vi "raster_scan_ground_shutter.vi"() -> ()   [LabVIEW 2013] (continued)
  out "Spectra":cluster{"X":dbl, "Y":dbl}[](graph)=[{"X"=497.2298226599585, "Y"=0.9725975182005102}, {"X"=498.51538166101153, "Y"=0.9728067925850153}, {"X"=499.8006653114716, "Y"=0.9747721051033233}, {"X"=501.08567369979005, "Y"=0.9751655628735649}, {"X"=502.37040691438784, "Y"=0.9732612176842215}, {"X"=503.65486504364054, "Y"=0.9746414011783826}, {"X"=504.9390481758954, "Y"=0.9742385776980085}, {"X"=506.2229563994542, "Y"=0.9735153291445955}, {"X"=507.50658980258396, "Y"=0.9733135229509433}, {"X"=508.7899484735106, "Y"=0.9744504839918318}, {"X"=510.0730325004275, "Y"=0.9766044345160604}, {"X"=511.3558419714845, "Y"=0.9750567839983721}, {"X"=512.6383769748013, "Y"=0.971673355532271}, {"X"=513.92063759845, "Y"=0.9740526614709577}, {"X"=515.2026239304761, "Y"=0.974130815359634}, {"X"=516.484336058878, "Y"=0.9752353326241979}, {"X"=517.7657740716236, "Y"=0.9733187917634595}, {"X"=519.0469380566371, "Y"=0.9738867743443941}, {"X"=520.3278281018086, "Y"=0.9741291463192384}, {"X"=521.6084442949887, "Y"=0.9739939491908779}, {"X"=522.8887867239932, "Y"=0.9738818697876678}, {"X"=524.1688554765973, "Y"=0.9751365110316095}, {"X"=525.448650640541, "Y"=0.9756894098172196}, {"X"=526.7281723035276, "Y"=0.9755958341013884}, {"X"=528.0074205532212, "Y"=0.9723731001887784}, {"X"=529.286395477245, "Y"=0.9736078210171095}, {"X"=530.5650971631895, "Y"=0.9753577492499681}, {"X"=531.8435256986106, "Y"=0.9756076345965283}, {"X"=533.1216811710165, "Y"=0.9749519370844743}, {"X"=534.3995636678867, "Y"=0.9737182292893943}, {"X"=535.6771732766625, "Y"=0.9731227772162603}, {"X"=536.954510084748, "Y"=0.9743263327011618}, {"X"=538.2315741795014, "Y"=0.9748905035101719}, {"X"=539.5083656482575, "Y"=0.9726015732101311}, {"X"=540.7848845783033, "Y"=0.9742346225867319}, {"X"=542.061131056891, "Y"=0.973702680791654}, {"X"=543.3371051712381, "Y"=0.9745816372249786}, {"X"=544.6128070085233, "Y"=0.9746140975084203}, {"X"=545.888236655888, "Y"=0.9745470905602152}, {"X"=547.1633942004373, "Y"=0.9740537792906223}, {"X"=548.438279729239, "Y"=0.9704166842457509}, {"X"=549.7128933293197, "Y"=0.9754447594924198}, {"X"=550.987235087676, "Y"=0.9748748689433028}, {"X"=552.261305091261, "Y"=0.9747804617231326}, {"X"=553.5351034269949, "Y"=0.9754642257486512}, {"X"=554.8086301817569, "Y"=0.9736484025754294}, {"X"=556.0818854423965, "Y"=0.9748432686352313}, {"X"=557.3548692957187, "Y"=0.9719628762042646}, {"X"=558.6275818284925, "Y"=0.9746558278490033}, {"X"=559.9000231274539, "Y"=0.9738137515041241}, {"X"=561.1721932793001, "Y"=0.9716527613161314}, {"X"=562.4440923706871, "Y"=0.974021060448881}, {"X"=563.7157204882404, "Y"=0.9728545916304719}, {"X"=564.9870777185446, "Y"=0.9732879649303774}, {"X"=566.2581641481513, "Y"=0.9744530162766258}, {"X"=567.5289798635712, "Y"=0.974627123784301}, {"X"=568.7995249512783, "Y"=0.9725287766595139}, {"X"=570.0697994977114, "Y"=0.9726663869699587}, {"X"=571.339803589273, "Y"=0.974955727849392}, {"X"=572.6095373123283, "Y"=0.9735543225094384}, {"X"=573.8790007532059, "Y"=0.9724127620578475}, {"X"=575.148193998193, "Y"=0.9740209723716318}, {"X"=576.4171171335469, "Y"=0.9735745739854244}, {"X"=577.6857702454895, "Y"=0.9736808497462064}, {"X"=578.9541534201954, "Y"=0.973725135201695}, {"X"=580.2222667438133, "Y"=0.9722570169385129}, {"X"=581.4901103024504, "Y"=0.9761561614512213}, {"X"=582.7576841821772, "Y"=0.9745066084652275}, {"X"=584.0249884690273, "Y"=0.9721193991121173}, {"X"=585.2920232489998, "Y"=0.9730164211590435}, {"X"=586.5587886080565, "Y"=0.9744353227462825}, {"X"=587.8252846321227, "Y"=0.9740001461801483}, {"X"=589.0915114070889, "Y"=0.9730116363864676}, {"X"=590.3574690188022, "Y"=0.9727604590195043}, {"X"=591.6231575530794, "Y"=0.9741329926815703}, {"X"=592.8885770957004, "Y"=0.9715013368639458}, {"X"=594.1537277324082, "Y"=0.9749212992460508}, {"X"=595.4186095489069, "Y"=0.9746155414778752}, {"X"=596.6832226308679, "Y"=0.9733153658733915}, {"X"=597.9475670639238, "Y"=0.9738269855570807}, {"X"=599.2116429336721, "Y"=0.9727047693027512}, {"X"=600.4754503256718, "Y"=0.9723284099559123}, {"X"=601.7389893254467, "Y"=0.9739548965405067}, {"X"=603.0022600184864, "Y"=0.9753519803682732}, {"X"=604.2652624902432, "Y"=0.9745724974660718}, {"X"=605.5279968261262, "Y"=0.9739205053321395}, {"X"=606.790463111523, "Y"=0.9733144490021569}, {"X"=608.0526614317708, "Y"=0.9736048889225003}, {"X"=609.3145918721773, "Y"=0.9737789504525353}, {"X"=610.5762545180146, "Y"=0.9755778166852583}, {"X"=611.8376494545141, "Y"=0.9730244273499707}, {"X"=613.0987767668724, "Y"=0.9728226921337769}, {"X"=614.3596365402559, "Y"=0.9752868467363005}, {"X"=615.6202288597873, "Y"=0.9735172698359681}, {"X"=616.8805538105571, "Y"=0.973124505522509}, {"X"=618.1406114776187, "Y"=0.9760376947254987}, {"X"=619.4004019459886, "Y"=0.9749446586217881}, {"X"=620.659925300649, "Y"=0.9727135962087332}, {"X"=621.9191816265427, "Y"=0.9769047701336491}, {"X"=623.1781710085843, "Y"=0.9737059369513906}, {"X"=624.4368935316431, "Y"=0.9730367708590156}, {"X"=625.6953492805558, "Y"=0.973595493502758}, {"X"=626.9535383401242, "Y"=0.9741996880818808}, {"X"=628.2114607951178, "Y"=0.9737205194986359}, {"X"=629.4691167302606, "Y"=0.9749579037936418}, {"X"=630.7265062302503, "Y"=0.9743079192507641}, {"X"=631.9836293797415, "Y"=0.9752794157731268}, {"X"=633.2404862633583, "Y"=0.9724798256913757}, {"X"=634.4970769656837, "Y"=0.9740631998947202}, {"X"=635.7534015712725, "Y"=0.9728994698167882}, {"X"=637.0094601646339, "Y"=0.9739938061766921}, {"X"=638.2652528302488, "Y"=0.9725288232542131}, {"X"=639.5207796525636, "Y"=0.9736153995992328}, {"X"=640.7760407159792, "Y"=0.9729825812921996}, {"X"=642.0310361048703, "Y"=0.9744619006373575}, {"X"=643.2857659035727, "Y"=0.9730632124324957}, {"X"=644.5402301963852, "Y"=0.9721840737194735}, {"X"=645.7944290675744, "Y"=0.974009871166903}, {"X"=647.0483626013629, "Y"=0.972528548755031}, {"X"=648.3020308819501, "Y"=0.9722772695955144}, {"X"=649.5554339934918, "Y"=0.976397196845756}, {"X"=650.8085720201068, "Y"=0.9735361483405925}, {"X"=652.0614450458858, "Y"=0.9743662972168945}, {"X"=653.3140531548762, "Y"=0.9733556726469628}, {"X"=654.5663964310929, "Y"=0.973308883274387}, {"X"=655.8184749585181, "Y"=0.9729671339680315}, {"X"=657.0702888210908, "Y"=0.9735267285897199}, {"X"=658.321838102726, "Y"=0.9736835283965779}, {"X"=659.5731228872934, "Y"=0.9724850110082932}, {"X"=660.8241432586319, "Y"=0.9768246153401708}, {"X"=662.0748993005419, "Y"=0.9747368444941559}, {"X"=663.3253910967932, "Y"=0.9748671054129099}, {"X"=664.5756187311121, "Y"=0.9712450801505587}, {"X"=665.8255822872012, "Y"=0.9733016295621294}, {"X"=667.0752818487133, "Y"=0.9751572607097476}, {"X"=668.3247174992814, "Y"=0.9736732199722962}, {"X"=669.5738893224913, "Y"=0.9714170347757555}, {"X"=670.8227974018998, "Y"=0.9744672290673195}, {"X"=672.0714418210257, "Y"=0.9735008611418889}, {"X"=673.3198226633544, "Y"=0.9753387615125017}, {"X"=674.5679400123306, "Y"=0.973086840492722}, {"X"=675.8157939513727, "Y"=0.9741838697202261}, {"X"=677.063384563856, "Y"=0.973529280298374}, {"X"=678.3107119331249, "Y"=0.9755250682367654}, {"X"=679.5577761424901, "Y"=0.9746411843678233}, {"X"=680.8045772752221, "Y"=0.9738103562180661}, {"X"=682.0511154145598, "Y"=0.9736968628203867}, {"X"=683.2973906437047, "Y"=0.9712589511537898}, {"X"=684.5434030458239, "Y"=0.9752582378141089}, {"X"=685.7891527040539, "Y"=0.976782251150417}, {"X"=687.0346397014858, "Y"=0.9731820071149043}, {"X"=688.2798641211891, "Y"=0.9733579906581664}, {"X"=689.5248260461898, "Y"=0.9744816274791854}, {"X"=690.769525559477, "Y"=0.9737516724400619}, {"X"=692.0139627440117, "Y"=0.9756854529656466}, {"X"=693.2581376827137, "Y"=0.9752736616888705}, {"X"=694.5020504584725, "Y"=0.9747129818582982}, {"X"=695.7457011541385, "Y"=0.9725964644867655}, {"X"=696.9890898525315, "Y"=0.9719206032188724}, {"X"=698.2322166364349, "Y"=0.975109207481176}, {"X"=699.4750815885972, "Y"=0.973770575651193}, {"X"=700.7176847917299, "Y"=0.9719288969600468}, {"X"=701.9600263285121, "Y"=0.9733333355442666}, {"X"=703.202106281586, "Y"=0.974777916241537}, {"X"=704.4439247335613, "Y"=0.9735484419792764}, {"X"=705.685481767011, "Y"=0.9717628831069969}, {"X"=706.9267774644752, "Y"=0.974585085670975}, {"X"=708.1678119084597, "Y"=0.9726989197644662}, {"X"=709.4085851814332, "Y"=0.9726006427385325}, {"X"=710.6490973658297, "Y"=0.9733097555076762}, {"X"=711.8893485440507, "Y"=0.9737219810572065}, {"X"=713.1293387984609, "Y"=0.9733159043764248}, {"X"=714.3690682113926, "Y"=0.974995019683123}, {"X"=715.6085368651409, "Y"=0.9744552200280534}, {"X"=716.8477448419642, "Y"=0.9728058762546018}, {"X"=718.0866922240972, "Y"=0.9737322943321336}, {"X"=719.3253790937289, "Y"=0.9735161803203743}, {"X"=720.5638055330157, "Y"=0.9730407067730923}, {"X"=721.8019716240839, "Y"=0.9709235684588909}, {"X"=723.0398774490205, "Y"=0.9745749775668794}, {"X"=724.2775230898802, "Y"=0.9744302526361133}, {"X"=725.5149086286827, "Y"=0.9723284652393392}, {"X"=726.7520341474134, "Y"=0.9753523975377738}, {"X"=727.9888997280249, "Y"=0.9750521852197641}, {"X"=729.2255054524308, "Y"=0.9745820478316395}, {"X"=730.4618514025187, "Y"=0.9742877083296526}, {"X"=731.6979376601308, "Y"=0.9751639925657974}, {"X"=732.933764307081, "Y"=0.976816750584068}, {"X"=734.1693314251528, "Y"=0.974162397219554}, {"X"=735.4046390960863, "Y"=0.9739741725110216}, {"X"=736.6396874015912, "Y"=0.9762852769993037}, {"X"=737.8744764233495, "Y"=0.9766708999836823}, {"X"=739.109006242997, "Y"=0.9753035240381733}, {"X"=740.343276942146, "Y"=0.975790884711858}, {"X"=741.5772886023653, "Y"=0.9766658088688991}, {"X"=742.8110413051957, "Y"=0.9785306717888759}, {"X"=744.0445351321432, "Y"=0.9760682422453827}, {"X"=745.2777701646746, "Y"=0.9780204446669288}, {"X"=746.5107464842309, "Y"=0.9782464109417868}, {"X"=747.7434641722119, "Y"=0.9772647154022579}, {"X"=748.9759233099848, "Y"=0.977692155970407}, {"X"=750.2081239788884, "Y"=0.9788852914399129}, {"X"=751.4400662602164, "Y"=0.9823419830408691}, {"X"=752.6717502352384, "Y"=0.9810201141633521}, {"X"=753.9031759851828, "Y"=0.9833986641137518}, {"X"=755.1343435912498, "Y"=0.9834070429804402}, {"X"=756.365253134605, "Y"=0.9825903876301169}, {"X"=757.5959046963706, "Y"=0.9839529209095583}, {"X"=758.8262983576512, "Y"=0.9813652342798371}, {"X"=760.0564341995022, "Y"=0.9844503443823484}, {"X"=761.2863123029542, "Y"=0.9839336674911496}, {"X"=762.5159327489974, "Y"=0.9850987306074251}, {"X"=763.7452956185957, "Y"=0.9859738872506251}, {"X"=764.9744009926738, "Y"=0.987104856944398}, {"X"=766.2032489521198, "Y"=0.986614152333766}, {"X"=767.4318395777977, "Y"=0.9923688895733606}, {"X"=768.6601729505263, "Y"=0.9903239765936077}, {"X"=769.8882491511001, "Y"=0.989832503713793}, {"X"=771.1160682602751, "Y"=0.9898834352980211}, {"X"=772.3436303587699, "Y"=0.9909275800922739}, {"X"=773.5709355272775, "Y"=0.9922316521951728}, {"X"=774.7979838464516, "Y"=0.9943163001250186}, {"X"=776.0247753969135, "Y"=0.9959180362878817}, {"X"=777.2513102592497, "Y"=0.9979176063076446}, {"X"=778.4775885140167, "Y"=0.997428897906833}, {"X"=779.7036102417335, "Y"=0.999946223134333}, {"X"=780.9293755228872, "Y"=0.9999233980339695}, {"X"=782.1548844379298, "Y"=1.001903497089305}, {"X"=783.3801370672809, "Y"=1.0032164241060768}, {"X"=784.6051334913254, "Y"=1.0017013431572122}, {"X"=785.8298737904138, "Y"=1.0042953210934331}, {"X"=787.0543580448677, "Y"=1.0057069045811273}, {"X"=788.2785863349704, "Y"=1.0040647666748501}, {"X"=789.5025587409746, "Y"=1.0051867459428807}, {"X"=790.7262753430958, "Y"=1.005057036199781}, {"X"=791.9497362215196, "Y"=1.0059360518630067}, {"X"=793.1729414563946, "Y"=1.008461102054222}, {"X"=794.3958911278411, "Y"=1.0087710728267973}, {"X"=795.6185853159403, "Y"=1.0112013829888278}, {"X"=796.8410241007414, "Y"=1.0111463852575098}, {"X"=798.0632075622646, "Y"=1.0110431430825668}, {"X"=799.2851357804917, "Y"=1.0112207906905948}, {"X"=800.5068088353718, "Y"=1.0108210325661546}, {"X"=801.7282268068236, "Y"=1.0109641328064574}, {"X"=802.9493897747267, "Y"=1.0130948150317125}, {"X"=804.1702978189347, "Y"=1.0119276625964746}, {"X"=805.3909510192625, "Y"=1.0117322027094646}, {"X"=806.6113494554919, "Y"=1.0104670902674695}, {"X"=807.8314932073748, "Y"=1.0125669362027019}, {"X"=809.0513823546283, "Y"=1.008923051883943}, {"X"=810.2710169769346, "Y"=1.0076251693882987}, {"X"=811.4903971539436, "Y"=1.0059566148313221}, {"X"=812.7095229652726, "Y"=1.0075916782638574}, {"X"=813.9283944905064, "Y"=1.0041324355776649}, {"X"=815.1470118091908, "Y"=1.0035018727995872}, {"X"=816.3653750008475, "Y"=1.0030209370577858}, {"X"=817.5834841449596, "Y"=0.999972510646731}, {"X"=818.8013393209794, "Y"=0.9982311340973924}, {"X"=820.0189406083226, "Y"=0.9980286387783647}, {"X"=821.2362880863745, "Y"=0.9966341239361585}, {"X"=822.453381834488, "Y"=0.993060330533325}, {"X"=823.6702219319809, "Y"=0.9917217165409767}, {"X"=824.8868084581368, "Y"=0.9904613412583302}, {"X"=826.1031414922085, "Y"=0.9890170518352254}, {"X"=827.3192211134187, "Y"=0.988833927457964}, {"X"=828.5350474009513, "Y"=0.9841303096381154}, {"X"=829.7506204339613, "Y"=0.9851113631293132}, {"X"=830.9659402915676, "Y"=0.9830141106198241}, {"X"=832.1810070528583, "Y"=0.9810835199593342}, {"X"=833.395820796889, "Y"=0.9802034001173303}, {"X"=834.6103816026787, "Y"=0.9793261517764306}, {"X"=835.8246895492179, "Y"=0.9794526534444457}, {"X"=837.0387447154625, "Y"=0.976711682992621}, {"X"=838.252547180336, "Y"=0.977505824867271}, {"X"=839.4660970227294, "Y"=0.976060708202824}, {"X"=840.6793943214965, "Y"=0.9775611768425274}, {"X"=841.8924391554654, "Y"=0.9779282090614275}, {"X"=843.1052316034272, "Y"=0.9749993032318836}, {"X"=844.3177717441384, "Y"=0.9766168015944888}, {"X"=845.5300596563252, "Y"=0.9770579025567279}, {"X"=846.7420954186853, "Y"=0.9761848317032691}, {"X"=847.9538791098754, "Y"=0.9750068893843726}, {"X"=849.1654108085241, "Y"=0.9766709018868858}, {"X"=850.3766905932297, "Y"=0.9762008333463423}, {"X"=851.587718542551, "Y"=0.9770669463188649}, {"X"=852.7984947350191, "Y"=0.9780283363764795}, {"X"=854.0090192491302, "Y"=0.9763912219061827}, {"X"=855.2192921633504, "Y"=0.9788411215148533}, {"X"=856.4293135561127, "Y"=0.9780523629858356}, {"X"=857.6390835058158, "Y"=0.9772591537506723}, {"X"=858.8486020908261, "Y"=0.9757138787241687}, {"X"=860.0578693894771, "Y"=0.9759727972704739}, {"X"=861.2668854800697, "Y"=0.9764995938198571}, {"X"=862.4756504408771, "Y"=0.9754531618170561}, {"X"=863.6841643501328, "Y"=0.9767196133220271}, {"X"=864.8924272860428, "Y"=0.9745194485252806}, {"X"=866.1004393267758, "Y"=0.9749240963153796}, {"X"=867.3082005504745, "Y"=0.9774754757373457}, {"X"=868.5157110352449, "Y"=0.9769089472275644}, {"X"=869.7229708591581, "Y"=0.9759113164154294}, {"X"=870.9299801002617, "Y"=0.975688860360333}, {"X"=872.1367388365617, "Y"=0.9755098405840466}, {"X"=873.3432471460362, "Y"=0.9774049464029454}, {"X"=874.5495051066284, "Y"=0.9766061555627099}, {"X"=875.7555127962536, "Y"=0.9791790276997551}, {"X"=876.9612702927898, "Y"=0.975348903104834}, {"X"=878.1667776740871, "Y"=0.9770138200310814}, {"X"=879.3720350179589, "Y"=0.976819345420831}, {"X"=880.5770424021898, "Y"=0.9774266354420642}, {"X"=881.7817999045305, "Y"=0.9770302925300669}, {"X"=882.9863076027008, "Y"=0.977857035396843}, {"X"=884.1905655743838, "Y"=0.9777987678144636}, {"X"=885.3945738972365, "Y"=0.9779807210693648}, {"X"=886.5983326488813, "Y"=0.9775173877335467}, {"X"=887.8018419069081, "Y"=0.9766485216340083}, {"X"=889.005101748874, "Y"=0.977437818767763}, {"X"=890.2081122523042, "Y"=0.9761858525398797}, {"X"=891.410873494695, "Y"=0.9746542684449129}, {"X"=892.613385553504, "Y"=0.9743258688686537}, {"X"=893.8156485061629, "Y"=0.9759803924600633}, {"X"=895.0176624300684, "Y"=0.9743203287756274}, {"X"=896.219427402587, "Y"=0.9780018850672363}, {"X"=897.4209435010506, "Y"=0.975819532988165}, {"X"=898.6222108027606, "Y"=0.9790767349064172}, {"X"=899.8232293849859, "Y"=0.977172571236749}, {"X"=901.023999324963, "Y"=0.9791890590838166}, {"X"=902.2245206998999, "Y"=0.9771201613401926}, {"X"=903.424793586966, "Y"=0.9754276213163193}, {"X"=904.6248180633042, "Y"=0.9766332088946419}, {"X"=905.8245942060255, "Y"=0.9755645009521582}, {"X"=907.0241220922055, "Y"=0.9778785245204034}, {"X"=908.2234017988899, "Y"=0.97618734926025}, {"X"=909.4224334030938, "Y"=0.9764876134860441}, {"X"=910.6212169817957, "Y"=0.9767751374191169}, {"X"=911.8197526119501, "Y"=0.9750979040027783}, {"X"=913.0180403704702, "Y"=0.976920621923853}, {"X"=914.2160803342456, "Y"=0.9742507611923987}, {"X"=915.4138725801308, "Y"=0.9751690344568648}, {"X"=916.6114171849462, "Y"=0.9756187195317623}, {"X"=917.8087142254856, "Y"=0.9764127552026054}, {"X"=919.0057637785084, "Y"=0.9758768475856276}, {"X"=920.2025659207393, "Y"=0.9785607427934253}, {"X"=921.3991207288747, "Y"=0.9753909084343684}, {"X"=922.5954282795807, "Y"=0.9756832948216083}, {"X"=923.7914886494865, "Y"=0.9770186365593877}, {"X"=924.9873019151955, "Y"=0.9780154929428406}, {"X"=926.1828681532783, "Y"=0.9773549557624684}, {"X"=927.3781874402686, "Y"=0.9737201953459799}, {"X"=928.5732598526744, "Y"=0.9776913581503284}, {"X"=929.7680854669686, "Y"=0.9765722632072701}, {"X"=930.9626643595965, "Y"=0.9775301787561222}, {"X"=932.1569966069658, "Y"=0.9774648517887062}, {"X"=933.3510822854564, "Y"=0.9775661602371771}, {"X"=934.5449214714181, "Y"=0.9757299850669123}, {"X"=935.7385142411698, "Y"=0.9763396913208743}, {"X"=936.9318606709917, "Y"=0.9751732518703343}, {"X"=938.124960837138, "Y"=0.9762385048279764}, {"X"=939.3178148158345, "Y"=0.9769355364789002}, {"X"=940.5104226832681, "Y"=0.9778265619579048}, {"X"=941.7027845155974, "Y"=0.9754004301194709}, {"X"=942.8949003889531, "Y"=0.9754185122899999}, {"X"=944.0867703794311, "Y"=0.975545568005335}, {"X"=945.2783945630944, "Y"=0.9777158690434975}, {"X"=946.4697730159781, "Y"=0.9744378227927594}, {"X"=947.6609058140851, "Y"=0.9764276916970946}, {"X"=948.851793033383, "Y"=0.9769308406202972}, {"X"=950.0424347498159, "Y"=0.9768353259937747}, {"X"=951.2328310392888, "Y"=0.9757398732413723}, {"X"=952.4229819776764, "Y"=0.9783109002089613}, {"X"=953.6128876408314, "Y"=0.9762623004632623}, {"X"=954.8025481045637, "Y"=0.9776791417025698}, {"X"=955.9919634446568, "Y"=0.9761067767179948}, {"X"=957.1811337368637, "Y"=0.9763600338979984}, {"X"=958.3700590569052, "Y"=0.9766313761596891}, {"X"=959.5587394804696, "Y"=0.9780148778733824}, {"X"=960.7471750832145, "Y"=0.9783881318304283}, {"X"=961.9353659407674, "Y"=0.9754049323214695}, {"X"=963.1233121287275, "Y"=0.977358218113531}, {"X"=964.3110137226596, "Y"=0.9763444634822267}, {"X"=965.4984707980932, "Y"=0.979519732600155}, {"X"=966.6856834305345, "Y"=0.9773106022529338}, {"X"=967.8726516954526, "Y"=0.9777624711863335}, {"X"=969.0593756682907, "Y"=0.9799532883528165}, {"X"=970.2458554244572, "Y"=0.9758132250505214}, {"X"=971.4320910393301, "Y"=0.979848459456216}, {"X"=972.618082588255, "Y"=0.9791074231403778}, {"X"=973.8038301465535, "Y"=0.9805743639785356}, {"X"=974.9893337895085, "Y"=0.9790169772769804}, {"X"=976.1745935923742, "Y"=0.9808698958868636}, {"X"=977.359609630375, "Y"=0.9814423007712825}, {"X"=978.5443819787, "Y"=0.9786045993284602}, {"X"=979.7289107125172, "Y"=0.9773087049878061}, {"X"=980.9131959069507, "Y"=0.9798944591362898}, {"X"=982.0972376371056, "Y"=0.9821217283875001}, {"X"=983.2810359780477, "Y"=0.9810317897396497}, {"X"=984.4645910048189, "Y"=0.9811456110048814}, {"X"=985.6479027924221, "Y"=0.9814657919085494}, {"X"=986.8309714158364, "Y"=0.9833586814302067}, {"X"=988.0137969500063, "Y"=0.9826333261152996}, {"X"=989.1963794698478, "Y"=0.9804090114789179}, {"X"=990.3787190502447, "Y"=0.9818180207058338}, {"X"=991.5608157660505, "Y"=0.982085255440518}, {"X"=992.7426696920857, "Y"=0.9828293936931858}, {"X"=993.9242809031451, "Y"=0.9832834049640772}, {"X"=995.1056494739889, "Y"=0.9820176582423806}, {"X"=996.286775479349, "Y"=0.9822903576469105}, {"X"=997.4676589939204, "Y"=0.9826636846390665}, {"X"=998.6483000923785, "Y"=0.9828654727686722}, {"X"=999.8286988493554, "Y"=0.9817220799810472}, {"X"=1001.008855339464, "Y"=0.9847798982223261}, {"X"=1002.1887696372777, "Y"=0.9830034859607621}, {"X"=1003.3684418173485, "Y"=0.9826558298259136}, {"X"=1004.5478719541869, "Y"=0.986346871778485}, {"X"=1005.7270601222801, "Y"=0.9843131014797006}, {"X"=1006.9060063960821, "Y"=0.9851045090481999}, {"X"=1008.0847108500193, "Y"=0.9837468737243986}, {"X"=1009.2631735584852, "Y"=0.9845773350315953}, {"X"=1010.4413945958407, "Y"=0.98351518774493}, {"X"=1011.6193740364213, "Y"=0.9852753993064831}, {"X"=1012.7971119545269, "Y"=0.9870847631024896}, {"X"=1013.9746084244323, "Y"=0.9857816047913267}, {"X"=1015.1518635203769, "Y"=0.9876554839515709}, {"X"=1016.3288773165722, "Y"=0.9833776098091495}, {"X"=1017.5056498871971, "Y"=0.984896704753769}, {"X"=1018.6821813064025, "Y"=0.9871878809592627}, {"X"=1019.8584716483109, "Y"=0.9886842590920442}, {"X"=1021.034520987008, "Y"=0.9872228983998851}, {"X"=1022.2103293965556, "Y"=0.9849583831909171}, {"X"=1023.3858969509809, "Y"=0.9870775875106531}, {"X"=1024.5612237242806, "Y"=0.9851725359534323}, {"X"=1025.7363097904279, "Y"=0.9857721995061369}, {"X"=1026.9111552233542, "Y"=0.9847213394602486}, {"X"=1028.085760096972, "Y"=0.9871714223523002}, {"X"=1029.2601244851523, "Y"=0.9839077158790588}, {"X"=1030.434248461751, "Y"=0.9848435560227394}, {"X"=1031.6081321005781, "Y"=0.984972713499061}, {"X"=1032.7817754754226, "Y"=0.9857785585046132}, {"X"=1033.9551786600382, "Y"=0.9849738738697786}, {"X"=1035.128341728155, "Y"=0.985021518022648}, {"X"=1036.3012647534665, "Y"=0.9835184165911383}, {"X"=1037.4739478096394, "Y"=0.9857324292093751}, {"X"=1038.6463909703068, "Y"=0.982808345481802}, {"X"=1039.8185943090791, "Y"=0.9813517320029487}, {"X"=1040.990557899526, "Y"=0.9833531134979133}, {"X"=1042.1622818151975, "Y"=0.9832699332691822}, {"X"=1043.3337661296073, "Y"=0.9815140117448664}, {"X"=1044.505010916242, "Y"=0.9839169634506533}, {"X"=1045.6760162485525, "Y"=0.9799492155918323}, {"X"=1046.8467821999673, "Y"=0.9787906981133734}, {"X"=1048.0173088438803, "Y"=0.9776854212899974}, {"X"=1049.1875962536571, "Y"=0.9794385669788094}, {"X"=1050.3576445026315, "Y"=0.9803808531174217}, {"X"=1051.5274536641123, "Y"=0.9780732659854674}, {"X"=1052.6970238113704, "Y"=0.9785644313731259}, {"X"=1053.8663550176543, "Y"=0.9801587703650743}, {"X"=1055.0354473561756, "Y"=0.9776050154342523}, {"X"=1056.204300900125, "Y"=0.975234918765309}, {"X"=1057.372915722651, "Y"=0.9769418042246533}, {"X"=1058.5412918968852, "Y"=0.9756550801276116}, {"X"=1059.7094294959227, "Y"=0.9755269653881015}, {"X"=1060.8773285928253, "Y"=0.9782573576373581}, {"X"=1062.0449892606337, "Y"=0.9770410463420607}, {"X"=1063.2124115723518, "Y"=0.9764147010868485}, {"X"=1064.379595600957, "Y"=0.9770932538888809}, {"X"=1065.5465414193943, "Y"=0.977463409585809}, {"X"=1066.713249100581, "Y"=0.9768480738384985}, {"X"=1067.8797187174075, "Y"=0.9755452152770404}, {"X"=1069.0459503427285, "Y"=0.9766336008802375}, {"X"=1070.2119440493693, "Y"=0.9759836590612925}, {"X"=1071.3776999101322, "Y"=0.9752569639241504}, {"X"=1072.5432179977843, "Y"=0.9765189492977305}, {"X"=1073.708498385063, "Y"=0.9777630588733446}, {"X"=1074.8735411446787, "Y"=0.9737696190560684}, {"X"=1076.0383463493079, "Y"=0.9749121436243413}, {"X"=1077.202914071603, "Y"=0.9762128250977328}, {"X"=1078.3672443841838, "Y"=0.9765420467860262}, {"X"=1079.5313373596398, "Y"=0.9761789312649787}, {"X"=1080.6951930705322, "Y"=0.9766068235229549}, {"X"=1081.8588115893901, "Y"=0.9746638171541231}, {"X"=1083.0221929887205, "Y"=0.9762718736360325}, {"X"=1084.185337340989, "Y"=0.9761945062135106}, {"X"=1085.3482447186423, "Y"=0.9753847953273749}, {"X"=1086.5109151940942, "Y"=0.9765190786761224}, {"X"=1087.673348839726, "Y"=0.9762149704904128}, {"X"=1088.835545727891, "Y"=0.9750405801160077}, {"X"=1089.997505930916, "Y"=0.977397805853606}, {"X"=1091.1592295210983, "Y"=0.9761023146775306}, {"X"=1092.3207165706972, "Y"=0.977320184327523}, {"X"=1093.4819671519535, "Y"=0.9744339672848474}, {"X"=1094.6429813370748, "Y"=0.9769480711869468}, {"X"=1095.8037591982345, "Y"=0.9764479785342535}, {"X"=1096.9643008075839, "Y"=0.9751379190329328}, {"X"=1098.124606237242, "Y"=0.9774455233284068}, {"X"=1099.2846755592975, "Y"=0.9757227905134439}, {"X"=1100.4445088458108, "Y"=0.9767591102990365}, {"X"=1101.604106168812, "Y"=0.9765533746427992}, {"X"=1102.7634676003006, "Y"=0.9772460994647658}, {"X"=1103.9225932122527, "Y"=0.9793188595601436}, {"X"=1105.081483076609, "Y"=0.9776478954163192}, {"X"=1106.240137265283, "Y"=0.9786257302448566}, {"X"=1107.3985558501593, "Y"=0.9755545136946714}, {"X"=1108.5567389030941, "Y"=0.9770400646362855}, {"X"=1109.714686495912, "Y"=0.9777222484450849}, {"X"=1110.872398700411, "Y"=0.9745043786751173}, {"X"=1112.0298755883584, "Y"=0.9785502183486503}, {"X"=1113.1871172314895, "Y"=0.9792697516983893}, {"X"=1114.344123701518, "Y"=0.9766185080299928}, {"X"=1115.5008950701201, "Y"=0.9790018921216935}, {"X"=1116.6574314089512, "Y"=0.9785756137032701}, {"X"=1117.8137327896288, "Y"=0.9776168793598988}, {"X"=1118.9697992837478, "Y"=0.9797148772422399}, {"X"=1120.1256309628714, "Y"=0.9768641535673591}, {"X"=1121.2812278985355, "Y"=0.9766260090777029}, {"X"=1122.4365901622411, "Y"=0.9794498042627646}, {"X"=1123.59171782547, "Y"=0.9787096646409332}, {"X"=1124.746610959668, "Y"=0.9818324577005738}, {"X"=1125.9012696362524, "Y"=0.9778366591131942}, {"X"=1127.0556939266132, "Y"=0.9782921073961083}, {"X"=1128.2098839021105, "Y"=0.980195206272053}, {"X"=1129.3638396340784, "Y"=0.9805784362071808}, {"X"=1130.517561193816, "Y"=0.9791144914489488}, {"X"=1131.6710486525988, "Y"=0.9792823895946341}, {"X"=1132.8243020816676, "Y"=0.9787146945429068}, {"X"=1133.9773215522457, "Y"=0.9778184975935033}, {"X"=1135.1301071355133, "Y"=0.978043485202979}, {"X"=1136.282658902633, "Y"=0.9808952101735956}, {"X"=1137.434976924733, "Y"=0.9771639732592449}, {"X"=1138.5870612729107, "Y"=0.9802243134912098}, {"X"=1139.73891201824, "Y"=0.9821837987356902}, {"X"=1140.89052923176, "Y"=0.980557279259247}, {"X"=1142.0419129844922, "Y"=0.9781236776112612}, {"X"=1143.1930633474153, "Y"=0.9797272440091299}, {"X"=1144.3439803914857, "Y"=0.9812316885291599}, {"X"=1145.4946641876345, "Y"=0.982274159992743}, {"X"=1146.6451148067595, "Y"=0.9769676606117542}, {"X"=1147.7953323197287, "Y"=0.9771363619802603}, {"X"=1148.9453167973836, "Y"=0.9795934257680596}, {"X"=1150.0950683105402, "Y"=0.9811310815018239}, {"X"=1151.2445869299772, "Y"=0.9801815354596745}, {"X"=1152.3938727264542, "Y"=0.9786047183146896}, {"X"=1153.5429257706958, "Y"=0.9790756585127013}, {"X"=1154.6917461334006, "Y"=0.9797441644494185}, {"X"=1155.8403338852388, "Y"=0.980861278242972}, {"X"=1156.988689096851, "Y"=0.9795955687933058}, {"X"=1158.1368118388468, "Y"=0.9781889893420528}, {"X"=1159.2847021818118, "Y"=0.9791738122304545}, {"X"=1160.4323601962997, "Y"=0.9803972823246944}, {"X"=1161.5797859528377, "Y"=0.9830298003921707}, {"X"=1162.7269795219252, "Y"=0.9786989779412593}, {"X"=1163.8739409740306, "Y"=0.9804163564281088}, {"X"=1165.0206703795948, "Y"=0.9800238730574915}, {"X"=1166.1671678090281, "Y"=0.979922308344655}, {"X"=1167.3134333327166, "Y"=0.9813249261736289}, {"X"=1168.4594670210145, "Y"=0.9784844096030403}, {"X"=1169.6052689442472, "Y"=0.9818457752707427}, {"X"=1170.750839172717, "Y"=0.9787884229698085}, {"X"=1171.8961777766926, "Y"=0.9807751536892163}, {"X"=1173.0412848264157, "Y"=0.9785234967317881}, {"X"=1174.1861603920988, "Y"=0.979300607959506}, {"X"=1175.3308045439246, "Y"=0.9786291107654863}, {"X"=1176.475217352054, "Y"=0.9793828810544655}, {"X"=1177.6193988866135, "Y"=0.9792778400457106}, {"X"=1178.7633492176983, "Y"=0.9773816698945632}, {"X"=1179.9070684153876, "Y"=0.9780522370934032}, {"X"=1181.0505565497203, "Y"=0.9771817230992123}, {"X"=1182.1938136907122, "Y"=0.980389779208075}, {"X"=1183.3368399083488, "Y"=0.9766641929961081}, {"X"=1184.479635272589, "Y"=0.9791154465658978}, {"X"=1185.6221998533638, "Y"=0.9760432563000407}, {"X"=1186.764533720574, "Y"=0.9750573613039952}, {"X"=1187.9066369440902, "Y"=0.9775283907535938}, {"X"=1189.048509593765, "Y"=0.9765119446540921}, {"X"=1190.1901517394103, "Y"=0.982490901212389}, {"X"=1191.3315634508142, "Y"=0.9774271577582775}, {"X"=1192.4727447977425, "Y"=0.9760373055117013}, {"X"=1193.6136958499228, "Y"=0.981729377288088}, {"X"=1194.7544166770629, "Y"=0.9773392802366685}, {"X"=1195.8949073488375, "Y"=0.9776325979578271}, {"X"=1197.0351679348917, "Y"=0.9775164071321929}, {"X"=1198.175198504853, "Y"=0.9768450334987449}, {"X"=1199.3149991283096, "Y"=0.9799860852770267}, {"X"=1200.454569874824, "Y"=0.9801756067511647}, {"X"=1201.593910813935, "Y"=0.9784046151621995}, {"X"=1202.7330220151507, "Y"=0.9770713797482681}, {"X"=1203.8719035479467, "Y"=0.9817049161155574}, {"X"=1205.010555481779, "Y"=0.9802169950740515}, {"X"=1206.1489778860691, "Y"=0.977958930725133}, {"X"=1207.287170830215, "Y"=0.9778365030902723}, {"X"=1208.4251343835836, "Y"=0.9768758935655317}, {"X"=1209.5628686155162, "Y"=0.9806572342396863}, {"X"=1210.7003735953217, "Y"=0.9826224773920289}, {"X"=1211.8376493922847, "Y"=0.9799837656433352}, {"X"=1212.974696075664, "Y"=0.9778173885940812}, {"X"=1214.1115137146862, "Y"=0.9793507492087162}, {"X"=1215.2481023785535, "Y"=0.9790345681864974}, {"X"=1216.3844621364337, "Y"=0.9829072532332083}, {"X"=1217.5205930574753, "Y"=0.9819228251184574}, {"X"=1218.6564952107958, "Y"=0.980263676576704}, {"X"=1219.7921686654809, "Y"=0.980198025050529}, {"X"=1220.927613490596, "Y"=0.9784785525753562}, {"X"=1222.0628297551707, "Y"=0.9812290528513234}, {"X"=1223.1978175282097, "Y"=0.9800765230074306}, {"X"=1224.3325768786945, "Y"=0.9795038575077939}, {"X"=1225.4671078755734, "Y"=0.9813762007206384}, {"X"=1226.6014105877698, "Y"=0.979476572194178}, {"X"=1227.7354850841757, "Y"=0.9794977097456937}, {"X"=1228.8693314336597, "Y"=0.9801943886781621}, {"X"=1230.002949705062, "Y"=0.9812966721772715}, {"X"=1231.1363399671905, "Y"=0.9812621464851005}, {"X"=1232.2695022888315, "Y"=0.9804823060619493}, {"X"=1233.4024367387426, "Y"=0.980221619481819}, {"X"=1234.5351433856472, "Y"=0.982707450493742}, {"X"=1235.6676222982492, "Y"=0.9821759166382027}, {"X"=1236.7998735452238, "Y"=0.9809159157852321}, {"X"=1237.9318971952143, "Y"=0.9808499582382387}, {"X"=1239.0636933168373, "Y"=0.980787144388752}, {"X"=1240.1952619786864, "Y"=0.9822617786598138}, {"X"=1241.326603249322, "Y"=0.9841497187360184}, {"X"=1242.4577171972787, "Y"=0.9817743900258021}, {"X"=1243.5886038910674, "Y"=0.9813837255303814}, {"X"=1244.7192633991658, "Y"=0.983242091127848}, {"X"=1245.8496957900265, "Y"=0.9820388375289683}, {"X"=1246.9799011320756, "Y"=0.9831536765275638}, {"X"=1248.1098794937134, "Y"=0.9811428827030896}, {"X"=1249.239630943305, "Y"=0.98091966482934}, {"X"=1250.3691555491946, "Y"=0.9801395827961259}, {"X"=1251.4984533796994, "Y"=0.9828352494934611}, {"X"=1252.6275245031072, "Y"=0.9830586412301664}, {"X"=1253.7563689876772, "Y"=0.9833162307150057}, {"X"=1254.8849869016424, "Y"=0.9823339989263119}, {"X"=1256.01337831321, "Y"=0.9811697943015885}, {"X"=1257.141543290557, "Y"=0.9826608197645347}, {"X"=1258.2694819018338, "Y"=0.9814902784141079}, {"X"=1259.3971942151677, "Y"=0.9836526717317958}, {"X"=1260.5246802986485, "Y"=0.9829688158439387}, {"X"=1261.6519402203512, "Y"=0.9818429119935838}, {"X"=1262.778974048316, "Y"=0.9835524929850067}, {"X"=1263.9057818505548, "Y"=0.978753642048282}, {"X"=1265.0323636950582, "Y"=0.9810342731602271}, {"X"=1266.1587196497815, "Y"=0.9837678033749649}, {"X"=1267.284849782663, "Y"=0.9823328941589646}, {"X"=1268.4107541616045, "Y"=0.9811139594321421}, {"X"=1269.536432854483, "Y"=0.9816377181225588}, {"X"=1270.6618859291505, "Y"=0.9808721551856653}, {"X"=1271.7871134534323, "Y"=0.980167103052229}, {"X"=1272.9121154951258, "Y"=0.9796446933481634}, {"X"=1274.0368921219979, "Y"=0.9819822087372755}, {"X"=1275.1614434017895, "Y"=0.9815475636461131}, {"X"=1276.2857694022202, "Y"=0.9820970427677869}, {"X"=1277.409870190974, "Y"=0.9813721952876066}, {"X"=1278.5337458357124, "Y"=0.9818064055971182}, {"X"=1279.6573964040692, "Y"=0.9796732119404893}, {"X"=1280.7808219636538, "Y"=0.9804189935917264}, {"X"=1281.904022582042, "Y"=0.9787924818212875}, {"X"=1283.0269983267906, "Y"=0.980918189835053}, {"X"=1284.1497492654194, "Y"=0.9781192135245974}, {"X"=1285.2722754654305, "Y"=0.978407056515436}, {"X"=1286.3945769942964, "Y"=0.9775316547798482}, {"X"=1287.5166539194583, "Y"=0.9794333917813969}, {"X"=1288.6385063083324, "Y"=0.9808655007710462}, {"X"=1289.7601342283147, "Y"=0.9789567383292009}, {"X"=1290.8815377467665, "Y"=0.9762498170354399}, {"X"=1292.0027169310238, "Y"=0.9752145568124546}, {"X"=1293.123671848393, "Y"=0.9769507916543909}, {"X"=1294.2444025661625, "Y"=0.9788811104888155}, {"X"=1295.3649091515833, "Y"=0.979968186304057}, {"X"=1296.4851916718885, "Y"=0.9768347743808443}, {"X"=1297.605250194275, "Y"=0.9815184163346751}, {"X"=1298.7250847859198, "Y"=0.9811704295355109}, {"X"=1299.844695513974, "Y"=0.9767446291205445}, {"X"=1300.9640824455569, "Y"=0.9783587988707628}, {"X"=1302.0832456477647, "Y"=0.9802571046232051}, {"X"=1303.2021851876618, "Y"=0.9786638089523889}, {"X"=1304.3209011322915, "Y"=0.9767594315364042}, {"X"=1305.4393935486657, "Y"=0.9789796662217214}, {"X"=1306.5576625037731, "Y"=0.9781812914793097}, {"X"=1307.6757080645762, "Y"=0.9790113242409225}, {"X"=1308.7935302980068, "Y"=0.9784729041379194}, {"X"=1309.9111292709715, "Y"=0.9795197705236592}, {"X"=1311.0285050503524, "Y"=0.9786609646125677}, {"X"=1312.1456577030035, "Y"=0.9818776733961269}, {"X"=1313.2625872957506, "Y"=0.9797178272572513}, {"X"=1314.3792938953916, "Y"=0.9794567802290707}, {"X"=1315.4957775687046, "Y"=0.9793161360773639}, {"X"=1316.6120383824332, "Y"=0.9778473862082161}, {"X"=1317.728076403301, "Y"=0.9784576237860806}, {"X"=1318.8438916979976, "Y"=0.9805314029343223}, {"X"=1319.959484333195, "Y"=0.9810455911004057}, {"X"=1321.074854375528, "Y"=0.977571900955021}, {"X"=1322.1900018916167, "Y"=0.9779357921007769}, {"X"=1323.3049269480418, "Y"=0.9771601028913797}, {"X"=1324.419629611369, "Y"=0.9811546297805358}, {"X"=1325.5341099481293, "Y"=0.9800806466047352}, {"X"=1326.6483680248343, "Y"=0.9778012794226257}, {"X"=1327.7624039079628, "Y"=0.9780119715879991}, {"X"=1328.8762176639677, "Y"=0.9780086692752783}, {"X"=1329.9898093592803, "Y"=0.9743639834978992}, {"X"=1331.1031790602992, "Y"=0.9796767730660833}, {"X"=1332.2163268334018, "Y"=0.9788934644352825}, {"X"=1333.3292527449364, "Y"=0.9753218510207314}, {"X"=1334.4419568612238, "Y"=0.9785220430156812}, {"X"=1335.5544392485633, "Y"=0.976917230725016}, {"X"=1336.666699973221, "Y"=0.9770629774045446}, {"X"=1337.7787391014397, "Y"=0.9778474916048328}, {"X"=1338.890556699438, "Y"=0.9793337677839182}, {"X"=1340.0021528334064, "Y"=0.9807324910362591}, {"X"=1341.1135275695074, "Y"=0.9807326440961897}, {"X"=1342.224680973875, "Y"=0.9768841658652381}, {"X"=1343.3356131126282, "Y"=0.9778004117508994}, {"X"=1344.446324051847, "Y"=0.9797938013111896}, {"X"=1345.5568138575918, "Y"=0.9790879372333942}, {"X"=1346.667082595893, "Y"=0.9785685204702061}, {"X"=1347.7771303327563, "Y"=0.9791810564623609}, {"X"=1348.8869571341645, "Y"=0.9783447901274761}, {"X"=1349.9965630660672, "Y"=0.9792375215348712}, {"X"=1351.1059481943928, "Y"=0.9791864199389575}, {"X"=1352.2151125850432, "Y"=0.9786485637383643}, {"X"=1353.3240563038926, "Y"=0.9801295491507578}, {"X"=1354.4327794167907, "Y"=0.9809143095707464}, {"X"=1355.5412819895575, "Y"=0.9779853793244822}, {"X"=1356.6495640879914, "Y"=0.978430242340626}, {"X"=1357.7576257778594, "Y"=0.9784902898937051}, {"X"=1358.865467124908, "Y"=0.9769971301031602}, {"X"=1359.9730881948528, "Y"=0.9794940879167484}, {"X"=1361.0804890533857, "Y"=0.9776985915834865}, {"X"=1362.1876697661744, "Y"=0.9818504927323705}, {"X"=1363.2946303988565, "Y"=0.9770204376039219}, {"X"=1364.401371017046, "Y"=0.9803210437777011}, {"X"=1365.5078916863283, "Y"=0.9779186375704139}, {"X"=1366.6141924722651, "Y"=0.9757973678810732}, {"X"=1367.720273440392, "Y"=0.9788554516447613}, {"X"=1368.826134656219, "Y"=0.9754435135671825}, {"X"=1369.9317761852228, "Y"=0.979209791944741}, {"X"=1371.03719809287, "Y"=0.9779956962937505}, {"X"=1372.1424004445857, "Y"=0.9801820832943918}, {"X"=1373.2473833057754, "Y"=0.9805113778365473}, {"X"=1374.3521467418184, "Y"=0.9784039643117454}, {"X"=1375.4566908180666, "Y"=0.9801892355050262}, {"X"=1376.5610155998493, "Y"=0.9782888543621753}, {"X"=1377.6651211524659, "Y"=0.9767919206148161}, {"X"=1378.7690075411917, "Y"=0.9777728867199803}, {"X"=1379.8726748312768, "Y"=0.9788222896700035}, {"X"=1380.976123087946, "Y"=0.975167883446235}, {"X"=1382.0793523763928, "Y"=0.9790037657192742}, {"X"=1383.1823627617907, "Y"=0.9823407897953931}, {"X"=1384.2851543092875, "Y"=0.980060318304625}, {"X"=1385.3877270839998, "Y"=0.9778054455071895}, {"X"=1386.4900811510236, "Y"=0.980245962263792}, {"X"=1387.592216575424, "Y"=0.9822243657828612}, {"X"=1388.6941334222483, "Y"=0.9792114959710196}, {"X"=1389.79583175651, "Y"=0.9800474934936249}, {"X"=1390.8973116432028, "Y"=0.9789482861612532}, {"X"=1391.9985731472877, "Y"=0.978924852675548}, {"X"=1393.0996163337081, "Y"=0.9815738884719079}, {"X"=1394.2004412673732, "Y"=0.9788828397369037}, {"X"=1395.301048013175, "Y"=0.9812596932707176}, {"X"=1396.401436635972, "Y"=0.9822312052737342}, {"X"=1397.5016072006042, "Y"=0.9829027257127224}, {"X"=1398.6015597718808, "Y"=0.9820282332623369}, {"X"=1399.7012944145854, "Y"=0.9827283925075851}, {"X"=1400.800811193479, "Y"=0.9819856540408946}, {"X"=1401.9001101732952, "Y"=0.9812051048010799}, {"X"=1402.9991914187412, "Y"=0.9835522666901612}, {"X"=1404.0980549945011, "Y"=0.9851208482757146}, {"X"=1405.1967009652274, "Y"=0.978468148116896}, {"X"=1406.2951293955582, "Y"=0.9843009323931298}, {"X"=1407.3933403500926, "Y"=0.9819390047769511}, {"X"=1408.4913338934164, "Y"=0.9822989907658619}, {"X"=1409.5891100900808, "Y"=0.9822484112133116}, {"X"=1410.6866690046133, "Y"=0.9841246368908421}, {"X"=1411.7840107015197, "Y"=0.9834804132733437}, {"X"=1412.8811352452772, "Y"=0.9810345216540809}, {"X"=1413.9780427003395, "Y"=0.9810293178021272}, {"X"=1415.0747331311302, "Y"=0.986332564502222}, {"X"=1416.1712066020527, "Y"=0.9879235762152561}, {"X"=1417.2674631774848, "Y"=0.9836972487890051}, {"X"=1418.3635029217742, "Y"=0.9843386379653614}, {"X"=1419.4593258992466, "Y"=0.9850021074218469}, {"X"=1420.554932174199, "Y"=0.9802550384908103}, {"X"=1421.6503218109099, "Y"=0.9824144898249717}, {"X"=1422.7454948736247, "Y"=0.9835321685063406}, {"X"=1423.8404514265694, "Y"=0.9862626051449139}, {"X"=1424.9351915339394, "Y"=0.9842445728767663}, {"X"=1426.0297152599087, "Y"=0.9860654012435021}, {"X"=1427.1240226686232, "Y"=0.9886547565869146}, {"X"=1428.2181138242047, "Y"=0.9838123116092378}, {"X"=1429.311988790751, "Y"=0.9812253957630864}, {"X"=1430.4056476323344, "Y"=0.9841697772387883}, {"X"=1431.4990904129966, "Y"=0.9823904592525758}, {"X"=1432.5923171967597, "Y"=0.9843129294620666}, {"X"=1433.6853280476196, "Y"=0.9821474169497116}, {"X"=1434.7781230295464, "Y"=0.9833049005999437}, {"X"=1435.8707022064846, "Y"=0.986638794866061}, {"X"=1436.9630656423537, "Y"=0.9826395310934701}, {"X"=1438.0552134010466, "Y"=0.9855129971321085}, {"X"=1439.147145546433, "Y"=0.9834688555716403}, {"X"=1440.2388621423574, "Y"=0.98413139234172}, {"X"=1441.3303632526383, "Y"=0.9844027621649721}, {"X"=1442.4216489410678, "Y"=0.9864459698557175}, {"X"=1443.5127192714142, "Y"=0.9827203910522815}, {"X"=1444.6035743074203, "Y"=0.9845162731205122}, {"X"=1445.6942141128043, "Y"=0.982881694760059}, {"X"=1446.7846387512611, "Y"=0.984481546455493}, {"X"=1447.874848286455, "Y"=0.9783034381591713}, {"X"=1448.9648427820287, "Y"=0.9800461234401086}, {"X"=1450.054622301601, "Y"=0.9834553236761199}, {"X"=1451.1441869087646, "Y"=0.9807275046564966}, {"X"=1452.2335366670843, "Y"=0.9809212174620677}, {"X"=1453.322671640105, "Y"=0.9838945763353488}, {"X"=1454.4115918913415, "Y"=0.979126965402405}, {"X"=1455.5002974842869, "Y"=0.9831514631741267}, {"X"=1456.5887884824083, "Y"=0.9801504200971485}, 
